vi "DAQmxTaskContainerConnect-Com-Exec.vi"(8 "error in (no error)":errorcluster, 9 "data":variant, 10 "ControlQueue":refnum<queue>, 11 "DAQmxTaskContainer in":refnum<class "DAQmxTaskContainer.lvclass">) -> (0 "error out":errorcluster, 3 "DAQmxTaskContainer out":refnum<class "DAQmxTaskContainer.lvclass">)   [LabVIEW 2015, in "DAQmxTaskContainer.lvclass"]
uses:
  DAQmxTaskContainer.lvclass
  dependecies/ControlsVIs/Clusters-def/DAQmx-Reply-Connect-client.ctl
  dependecies/ControlsVIs/Clusters-def/DAQmx-Reply-to-Connect.ctl
  dependecies/ControlsVIs/Clusters-def/SERVER-Commands.ctl
  DAQmxTask.lvclass
  Control/Control-Server/Control-Server.lvclass
  DAQmxTaskContainer_General/DAQmxTaksContainer_General.lvclass
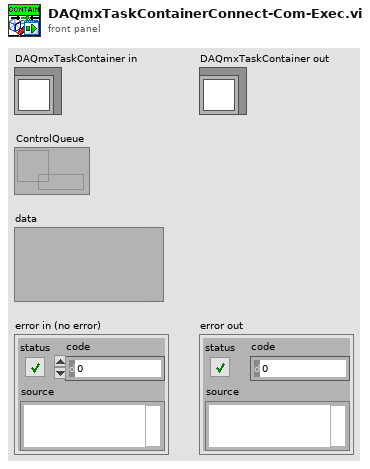
[diagram p1: front panel]
types:
  T1 = typedef "Control-Server.lvclass/SERVER-Commands.ctl" = string
  T2 = typedef "DAQmxTaksContainer_General.lvclass/DAQmx-Reply-to-Connect.ctl" = cluster{"On/Off":bool, "error":errorcluster, "DAQmxTaskContainer":refnum<class "DAQmxTaskContainer.lvclass">}
  T3 = typedef "DAQmxTaksContainer_General.lvclass/DAQmx-Reply-Connect-client.ctl" = cluster{"on/off":bool, "RelayKeyHeater/off":bool, "LaserShutter":bool, "AcceleratorShutter":bool, "Power":bool, "Faraday Cup Status":bool, "error":errorcluster}
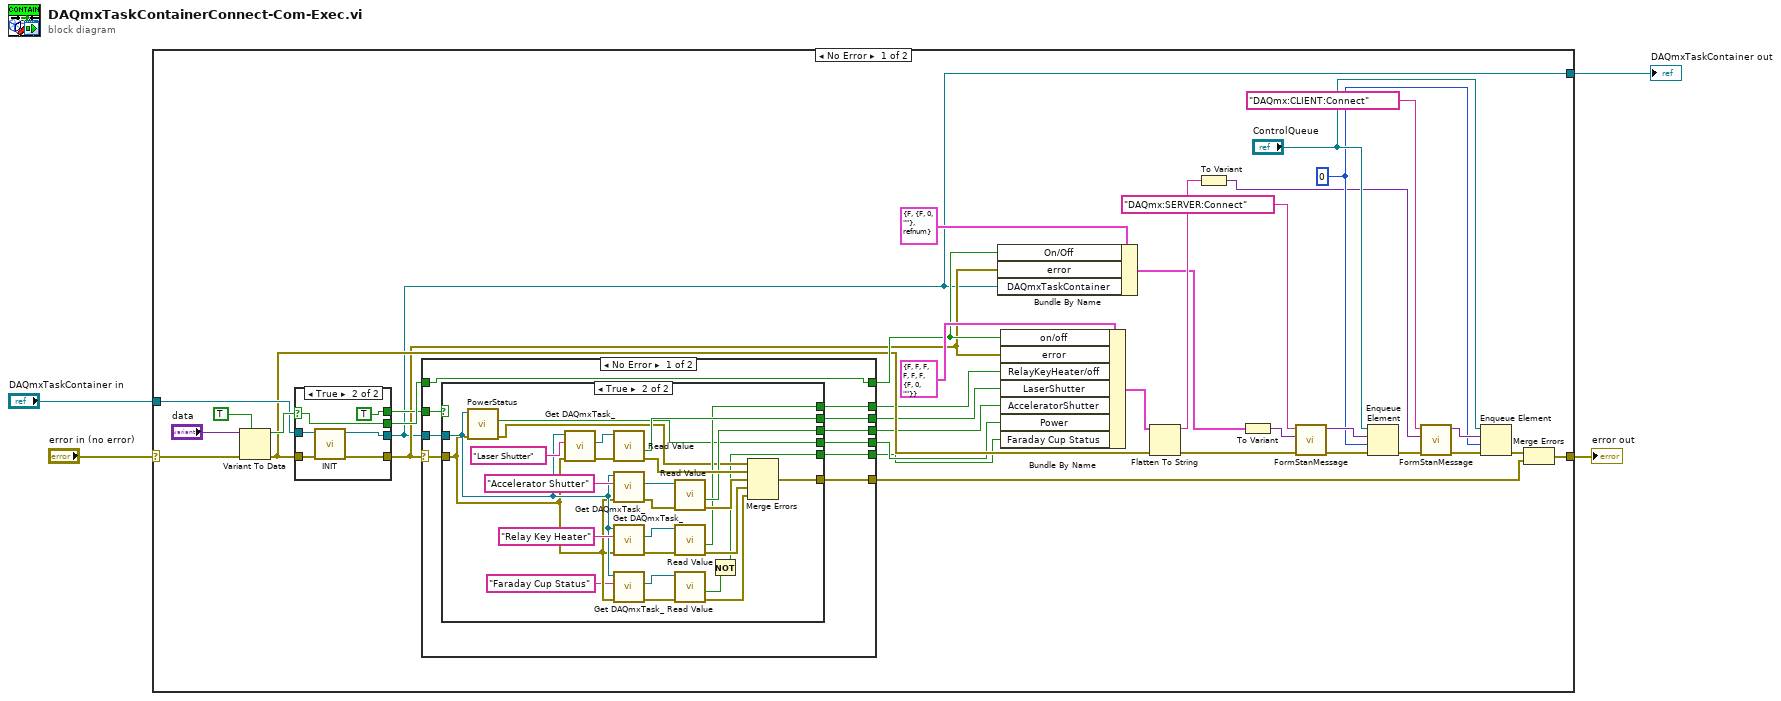
[diagram p0: block diagram]
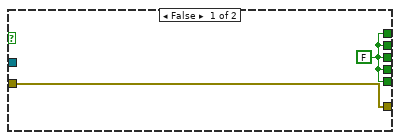
[diagram p2: hidden frame]
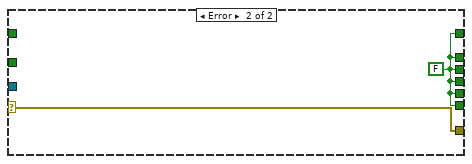
[diagram p3: hidden frame]
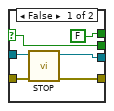
[diagram p4: hidden frame]
diagram:
  n1 = case shown="No Error" "error in (no error)" {
    selector: "error in (no error)" -> [w31 w94]
    tunnel: [w30 w94] -> w4
    tunnel: "DAQmxTaskContainer in" -> [w29 w93]
    tunnel: [w16 w93] -> w2
    frame No Error {
      w8 = 0 ("timeout en ms (-1)")
      n2 = Variant To Data(error in=w31, type=TRUE, Variant="data") -> (data=w38:bool, error out=w28:errorcluster)
      n3 = case shown="True" w38 {
        selector: w38 -> [w83 w89]
        tunnel: w29 -> [w86 w92]
        tunnel: [w85 w91] -> w16
        tunnel: [w84 w90] -> w17
        tunnel: [w83 w89] -> w37
        tunnel: w28 -> [w81 w88]
        tunnel: [FALSE TRUE] -> w27
        frame False {
          n4 = call-dynamic "STOP.vi"("error in (no error)"=w81, "DAQmxTaskContainer en entrée"=w86) -> ("error out"=w84:errorcluster, "DAQmxTaskContainer en sortie"=w85:refnum<class "DAQmxTaskContainer.lvclass">)  [unwired: 8 in]
        }
        frame True {
          n5 = call-dynamic "INIT.vi"("error in (no error)"=w88, "DAQmxTaskContainer en entrée"=w92) -> ("error out"=w90:errorcluster, "DAQmxTaskContainer en sortie"=w91:refnum<class "DAQmxTaskContainer.lvclass">)  [unwired: 8 in]
        }
      }
      n6 = case shown="No Error" w17 {
        selector: w17 -> [w47 w80]
        tunnel: [w50 w79] -> w32
        tunnel: w37 -> [w50 _]
        tunnel: w27 -> [w49 _]
        tunnel: w16 -> [w48 _]
        tunnel: [w46 w80] -> w26
        tunnel: [w45 w79] -> w25
        tunnel: [w44 w79] -> w24
        tunnel: [w43 w79] -> w23
        tunnel: [w42 w79] -> w22
        tunnel: [w41 w79] -> w21
        frame No Error {
          n7 = case shown="True" w49 {
            tunnel: w48 -> [_ w56]
            tunnel: w47 -> [w52 w55]
            tunnel: [w52 w66] -> w46
            tunnel: [w51 w61] -> w45
            tunnel: [w51 w65] -> w44
            tunnel: [w51 w64] -> w43
            tunnel: [w51 w63] -> w42
            tunnel: [w51 w53] -> w41
            frame False {
              w51 = FALSE ("Data")
            }
            frame True {
              n8 = call "PowerStatus.vi"("error in (no error)"=w55, "DAQmxTaskContainer in"=w56) -> ("error out"=w62:errorcluster, "On/Off"=w61:bool)  [unwired: 7 in, 1 out]
              n9 = call "Get DAQmxTask_.vi"("error in (no error)"=w55, "Task name"="Laser Shutter", "DAQmxTaksContainer_General in"=w56) -> ("error out"=w70:errorcluster, "DAQmx Task"=w71:refnum<class "DAQmxTask.lvclass">)  [unwired: 6 in, 1 out]
              n10 = call-dynamic "Read Value.vi"("error in (no error)"=w70, "DAQmxTask en entrée"=w71) -> ("error out"=w76:errorcluster, "Data"=w65:bool)  [unwired: 6 in, 2 out]
              n11 = call "Get DAQmxTask_.vi"("error in (no error)"=w55, "Task name"="Accelerator Shutter", "DAQmxTaksContainer_General in"=w56) -> ("error out"=w72:errorcluster, "DAQmx Task"=w73:refnum<class "DAQmxTask.lvclass">)  [unwired: 6 in, 1 out]
              n12 = call "Get DAQmxTask_.vi"("error in (no error)"=w55, "Task name"="Relay Key Heater", "DAQmxTaksContainer_General in"=w56) -> ("error out"=w74:errorcluster, "DAQmx Task"=w75:refnum<class "DAQmxTask.lvclass">)  [unwired: 6 in, 1 out]
              n13 = call "Get DAQmxTask_.vi"("error in (no error)"=w55, "Task name"="Faraday Cup Status", "DAQmxTaksContainer_General in"=w56) -> ("error out"=w58:errorcluster, "DAQmx Task"=w57:refnum<class "DAQmxTask.lvclass">)  [unwired: 6 in, 1 out]
              n14 = call-dynamic "Read Value.vi"("error in (no error)"=w72, "DAQmxTask en entrée"=w73) -> ("error out"=w77:errorcluster, "Data"=w64:bool)  [unwired: 6 in, 2 out]
              n15 = call-dynamic "Read Value.vi"("error in (no error)"=w74, "DAQmxTask en entrée"=w75) -> ("error out"=w78:errorcluster, "Data"=w63:bool)  [unwired: 6 in, 2 out]
              n16 = call-dynamic "Read Value.vi"("error in (no error)"=w58, "DAQmxTask en entrée"=w57) -> ("error out"=w60:errorcluster, "Data"=w59:bool)  [unwired: 6 in, 2 out]
              n17 = Not(x=w59) -> (.not. x?=w53:bool)
              n18 = Merge Errors(w62, w76, w77, w78, w60) -> (w66:errorcluster)
            }
          }
        }
        frame Error {
          w79 = FALSE
        }
      }
      n19 = Bundle By Name(cluster=T2 {"On/Off"=FALSE, "error"={"status"=FALSE, "code"=0, "source"=""}, "DAQmxTaskContainer"=refnum} ("Cluster"), "On/Off"=w32, "error"=w17, "DAQmxTaskContainer"=w16) -> (w6:T2)
      n20 = Bundle By Name(cluster=T3 {"on/off"=FALSE, "RelayKeyHeater/off"=FALSE, "LaserShutter"=FALSE, "AcceleratorShutter"=FALSE, "Power"=FALSE, "Faraday Cup Status"=FALSE, "error"={"status"=FALSE, "code"=0, "source"=""}} ("output cluster"), "on/off"=w32, "error"=w17, "RelayKeyHeater/off"=w22, "LaserShutter"=w24, "AcceleratorShutter"=w23, "Power"=w25, "Faraday Cup Status"=w21) -> (w35:T3)
      n21 = Flatten To String(anything=w35, error in (no error)=w28) -> (data string=w34:string, error out=w5:errorcluster)  [unwired: 2 in, 1 out]
      n22 = To Variant(anything=w34) -> (Variant=w7:variant)
      n23 = To Variant(anything=w6) -> (Variant=w14:variant)
      n24 = call "FormStanMessage.vi"("error in"=w5, "data"=w14, "Command"=T1 "DAQmx:SERVER:Connect" ("Commands")) -> ("error out"=w20:errorcluster, "message"=w19:variant)  [unwired: 7 in]
      n25 = Enqueue Element(queue="ControlQueue", element=w19, timeout in ms (-1)=w8, error in (no error)=w20) -> (error out=w11:errorcluster)  [unwired: 2 out]
      n26 = call "FormStanMessage.vi"("error in"=w11, "data"=w7, "Command"=T1 "DAQmx:CLIENT:Connect" ("Commands")) -> ("error out"=w12:errorcluster, "message"=w13:variant)  [unwired: 7 in]
      n27 = Enqueue Element(queue="ControlQueue", element=w13, timeout in ms (-1)=w8, error in (no error)=w12) -> (error out=w10:errorcluster)  [unwired: 2 out]
      n28 = Merge Errors(w10, w26) -> (w30:errorcluster)
    }
    frame Error {
    }
  }
  "error out" <- w4
  "DAQmxTaskContainer out" <- w2
